vi "Parse Comment.vi"(8 "Error In":errorcluster) -> (0 "Error Out":errorcluster)   [LabVIEW 2018, in "Tests.lvlib" / "Lexer.lvlib"]
uses:
  Lexer.lvlib
  src/Toolkit/Low-Level/Tokens/Comment/Comment.lvclass
  src/Toolkit/Low-Level/Support/Lex String.vi
  <vilib>/Utility/LVClass/Get LV Class Name.vi
  src/Toolkit/Low-Level/Tokens/Contentable/Contentable.lvclass
  <vilib>/addons/_JKI Toolkits/Caraya/classes/Test/Test.lvclass
  <vilib>/addons/_JKI Toolkits/Caraya/classes/Assert/Assert.lvclass
  src/Toolkit/Toolkit.lvlib
  Tests.lvlib
  src/Toolkit/Low-Level/Tokens/Abstract/Abstract.lvclass
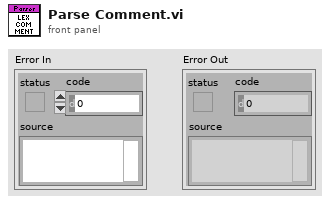
[diagram p1: front panel]
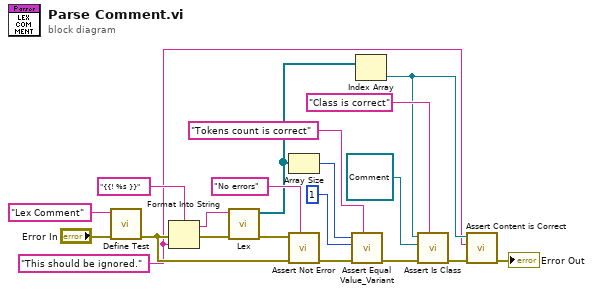
[diagram p0: block diagram]
diagram:
  w1 = "This should be ignored." ("format string")
  n1 = call <vilib>:"Define Test.vi"("error in (no error)"="Error In", "Label (VI Title)"="Lex Comment") -> ("error out"=w12:errorcluster)  [unwired: 9 in]
  n2 = Format Into String(format string="{{! %s }}", error in=w12, w1) -> (resulting string=w2:string, error out=w4:errorcluster)  [unwired: 1 in]
  n3 = call-poly "Lex.vi"("Error In"=w4, "Input"=w2) -> ("Error Out"=w18:errorcluster, "Tokens"=w9:refnum<class "Abstract.lvclass">[])  [unwired: 8 in]
  n4 = Array Size(array=w9) -> (size(s)=w14:i32)
  n5 = call <vilib>:"Assert Not Error.vi"("Label"="No errors", "error in (no error)"=w12, "Not Error?"=w18) -> ("error out"=w16:errorcluster)  [unwired: 8 in]
  n6 = call <vilib>:"Assert Equal Value_Variant.vi"("Label"="Tokens count is correct", "error in (no error)"=w16, "Y"=1 ("size(s)"), "X"=w14) -> ("error out"=w11:errorcluster)  [unwired: 7 in]
  n7 = Index Array(array=w9) -> (element=w5:refnum<class "Abstract.lvclass">)  [unwired: 1 in]
  n8 = call "Assert Is Class.vi"("Label"="Class is correct", "Error In"=w11, "Expected"=refnum<class "Comment.lvclass"> refnum ("Toolkit.lvlib:Tokens.lvlib:Comment.lvclass"), "Actual"=w5) -> ("Error Out"=w10:errorcluster)  [unwired: 7 in]
  n9 = call "Assert Content is Correct.vi"("Error In"=w10, "Expected"=w1, "Token"=w5) -> ("Error Out"=→"Error Out":errorcluster)  [unwired: 8 in]
